vi "Integration.vi"(9 "dt":dbl, 10 "x_dot":dbl, 11 "x(n-1)":dbl) -> (3 "x(n)":dbl)   [LabVIEW 2017]
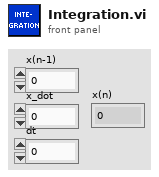
[diagram p1: front panel]
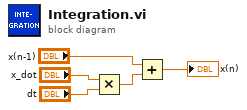
[diagram p0: block diagram]
diagram:
  n1 = Multiply(x="x_dot", y="dt") -> (x*y=w2:dbl)
  n2 = Add(x="x(n-1)", y=w2) -> (x+y=→"x(n)":dbl)
